vi "orig folder file list and path.vi"(8 "error in":errorcluster, 11 "path_Orig":path) -> (0 "error out":errorcluster, 3 "cl_filename_pathout":T1(array[cluster]))   [LabVIEW 2026]
doc: "This subVI checks original folder and obtains all files and information"
panel:
  out "arr_pathout":path[](array[path])
  out "path out":path
  out "filenames":string[](array[string])
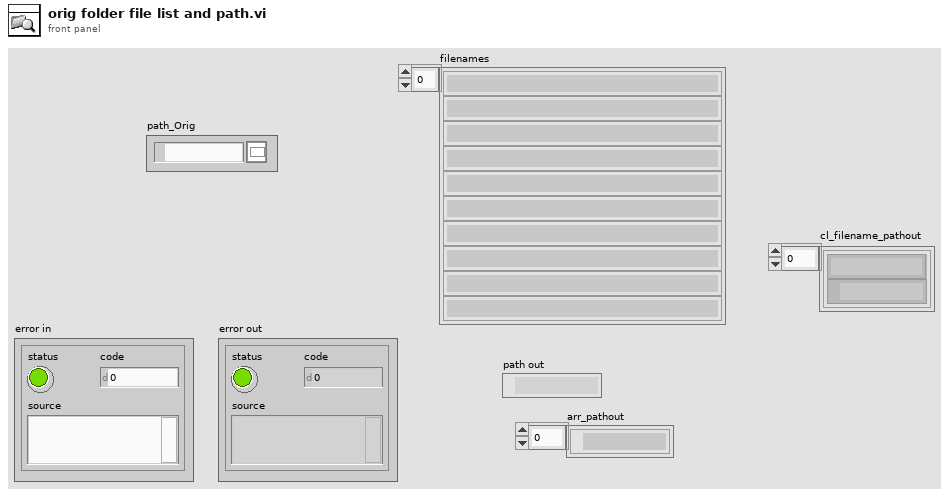
[diagram p1: front panel]
types:
  T1 = cluster{"filename":string, "arr_path out 2":path}[]
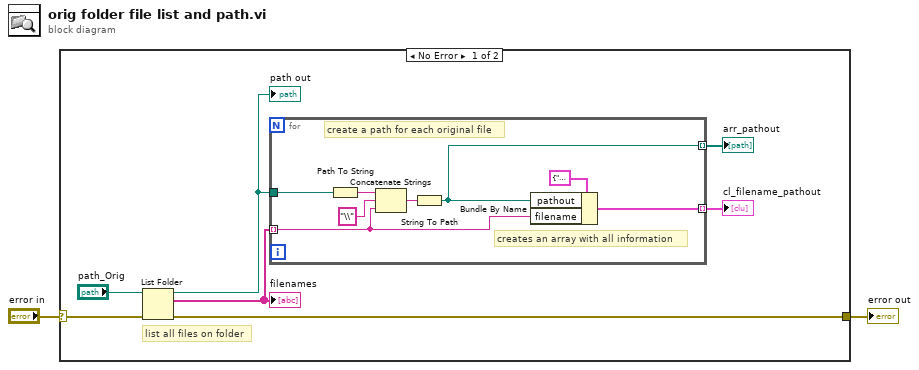
[diagram p0: block diagram]
diagram:
  n1 = case shown="No Error" "error in" {
    selector: "error in" -> [w8 w18]
    tunnel: [w7 w18] -> w1
    frame No Error {
      # "list all files on folder"
      n2 = List Folder(path="path_Orig", error in=w8) -> (path out=w5:path, filenames=w6:string[], error out=w7:errorcluster)  [unwired: 1 in, 2 out]
      "filenames" <- w6
      "path out" <- w5
      n3 = for {
        tunnel: w6 -> [w10] mode=indexing
        tunnel: w5 -> [w17]
        tunnel: [w11] -> w4 mode=indexing
        tunnel: [w12] -> w3 mode=indexing
        # "creates an array with all information"
        # "create a path for each original file"
        n4 = Path To String(path=w17) -> (string=w15:string)
        n5 = Concatenate Strings(w15, "\\", w10) -> (w16:string)
        n6 = String To Path(string=w16) -> (path=w11:path)
        n7 = Bundle By Name(cluster=cluster{"filename":string, "pathout":path} {"filename"="", "pathout"=path ""} ("cl_filename_pathout"), "pathout"=w11, "filename"=w10) -> (w12:cluster{"filename":string, "pathout":path})
      }
      "arr_pathout" <- w4
      "cl_filename_pathout" <- w3
    }
    frame Error {
    }
  }
  "error out" <- w1
